vi "Set Dev Notice Call Back.vi"(9 "rmvcallback":cluster{}, 10 "addcallback":cluster{}, 11 "ppara":u32) -> (3 "ppara out":u32)   [LabVIEW 2021, in "vmmso.lvlib"]
doc: "DLL_API void WINAPI SetDevNoticeCallBack(void* ppara, AddCallBack addcallback, RemoveCallBack rmvcallback);"
uses:
  vmmso.lvlib
  vmmso.dll
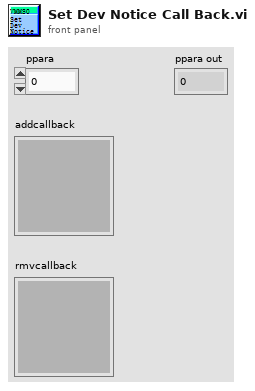
[diagram p1: front panel]
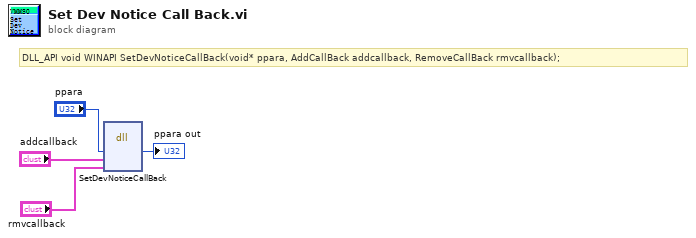
[diagram p0: block diagram]
diagram:
  # "DLL_API void WINAPI SetDevNoticeCallBack(void* ppara, AddCallBack addcallback, RemoveCallBack rmvcallback);"
  n1 = dll-call lib="D:/labviewdemo/LabviewDemo 21/vmmso/vmmso.*" fn="SetDevNoticeCallBack"("ppara"="ppara", "addcallback"="addcallback", "rmvcallback"="rmvcallback") -> ("ppara"=→"ppara out":u32)  [unwired: 6 in, 2 out]
